vi "LoadParser.vi"(4 "PythonPath":path, 6 "PythonVersion":string, 7 "SessionName":string, 8 "error in (no error)":errorcluster, 10 "ParserPath":path, 11 "ModulePath":path) -> (0 "error out":errorcluster, 3 "ArgumentParser":refnum<class "ArgumentParser.lvclass">)   [LabVIEW 2022 SP3, in "ArgumentParser.lvlib" / "ArgumentParser.lvclass"]
uses:
  ArgumentParser.lvclass
  C:/Users/jakub/repos/gh/sw4sys/lv-argument-parser/PythonWrapper/Source/PythonSession/PythonSession.lvclass
  C:/Users/jakub/repos/gh/sw4sys/lv-argument-parser/PythonWrapper/Source/PythonWrapper/PythonWrapper.lvclass
  C:/Users/jakub/repos/gh/sw4sys/lv-argument-parser/ArgumentParser/Source/ArgparseWrapper/ArgparseWrapper.lvclass
  PythonWrapper/Source/PythonSession/PythonSession.lvclass/PythonSession.ctl
  PythonWrapper/Source/PythonWrapper/PythonWrapper.lvclass/PythonWrapper.ctl
  ArgparseWrapper/ArgparseWrapper.lvclass/ArgparseWrapper.ctl
  ArgumentParser.lvclass/ArgumentParser.ctl
  PythonWrapper/Source/PythonSession/Write SessionName.vi
  PythonWrapper/Source/PythonSession/Write PythonVersion.vi
  PythonWrapper/Source/PythonSession/Write PythonPath.vi
  PythonWrapper/Source/PythonWrapper/Write ModulePath.vi
  PythonWrapper/Source/PythonSession/Read PythonSession.vi
  PythonWrapper/Source/PythonWrapper/Read ModulePath.vi
  Read Parser.vi
  Write Parser.vi
  PathUtils/Source/PathUtils.lvlib
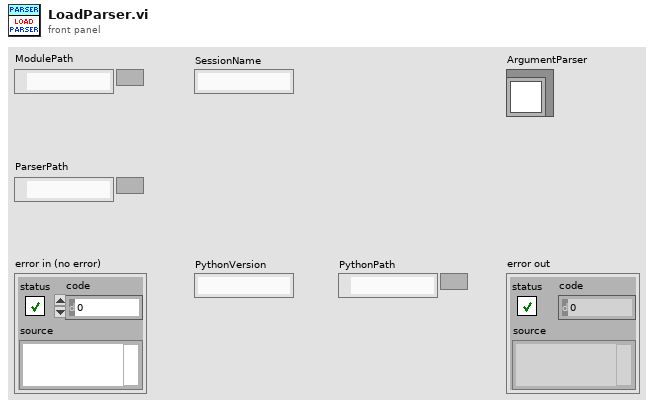
[diagram p1: front panel]
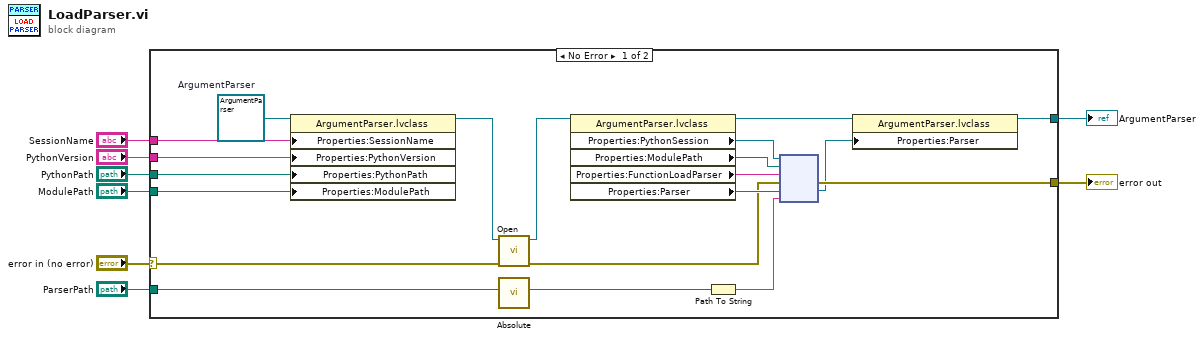
[diagram p0: block diagram]
diagram:
  n1 = case shown="No Error" "error in (no error)" {
    selector: "error in (no error)" -> [w27 w29]
    tunnel: [w28 w29] -> w7
    tunnel: [w25 _] -> w6
    tunnel: "ModulePath" -> [w13 _]
    tunnel: "ParserPath" -> [w18 _]
    tunnel: "PythonVersion" -> [w15 _]
    tunnel: "PythonPath" -> [w14 _]
    tunnel: "SessionName" -> [w12 _]
    frame No Error {
      w16 = refnum<class "ArgumentParser.lvclass"> refnum  # ArgumentParser
      n2 = property class="ArgumentParser.lvclass"(reference=w16, "Properties:SessionName"=w12, "Properties:PythonVersion"=w15, "Properties:PythonPath"=w14, "Properties:ModulePath"=w13) -> (reference out=w11:refnum<class "ArgumentParser.lvclass">)  [unwired: 1 in, 1 out]
      n3 = call-dynamic "Open.vi"("error in (no error)"=w27, "PythonWrapper in"=w11) -> ("error out"=w19:errorcluster, "PythonWrapper out"=w10:refnum<class "ArgumentParser.lvclass">)  [unwired: 8 in]
      n4 = call "Absolute.vi"("Path in"=w18) -> ("Path out"=w9:path)  [unwired: 10 in]
      n5 = property class="ArgumentParser.lvclass"(reference=w10) -> (reference out=w24:refnum<class "ArgumentParser.lvclass">, "Properties:PythonSession"=w22:refnum<k35>, "Properties:ModulePath"=w21:path, "Properties:FunctionLoadParser"=w23:string, "Properties:Parser"=w20:refnum<k38>)  [unwired: 1 in, 1 out]
      n6 = Path To String(path=w9) -> (string=w17:string)
      n7 = node(w22, w21, w23, w19, w20, w17) -> (w28:errorcluster, w26:refnum<k38>)  [unwired: 1 in, 3 out]
      n8 = property class="ArgumentParser.lvclass"(reference=w24, "Properties:Parser"=w26) -> (reference out=w25:refnum<class "ArgumentParser.lvclass">)  [unwired: 1 in, 1 out]
    }
    frame Error {
    }
  }
  "error out" <- w7
  "ArgumentParser" <- w6
